vi "AlazarTriggered.vi"(0 "Handle":u64, 1 "error in (no error)":errorcluster) -> (2 "Handle":u64, 3 "Triggered":bool, 5 "error out":errorcluster)   [LabVIEW 2009]
doc: "Determine if a board has triggered during the current acquisition."
uses:
  ATSApi.dll
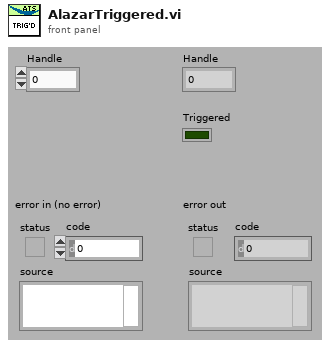
[diagram p1: front panel]
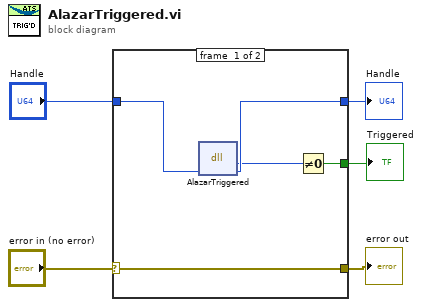
[diagram p0: block diagram]
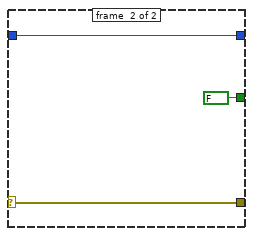
[diagram p2: hidden frame]
diagram:
  n1 = case shown="No Error" "error in (no error)" {
    selector: "error in (no error)" -> [w8 w13]
    tunnel: [w8 w13] -> w4
    tunnel: "Handle" -> [w10 w12]
    tunnel: [w9 w12] -> w2
    tunnel: [w6 FALSE] -> w1
    frame #0 {
      n2 = dll-call lib="ATSApi.dll" fn="AlazarTriggered"("handle"=w10) -> ("return type"=w7:u32, "handle"=w9:u64)  [unwired: 3 in, 2 out]
      n3 = Not Equal To 0?(x=w7) -> (x != 0?=w6:bool)
    }
    frame #1 {
    }
  }
  "Handle" <- w2
  "error out" <- w4
  "Triggered" <- w1
